vi "a20240618-1.vi"() -> ()   [LabVIEW 2019]
panel:
  out "Array":dbl[](array[numeric])
  out "Numeric 4":dbl
  out "Numeric 3":dbl
  out "Numeric 2":dbl
  in  "stop":bool
  out "Numeric":dbl
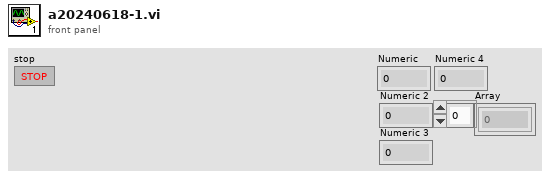
[diagram p1: front panel]
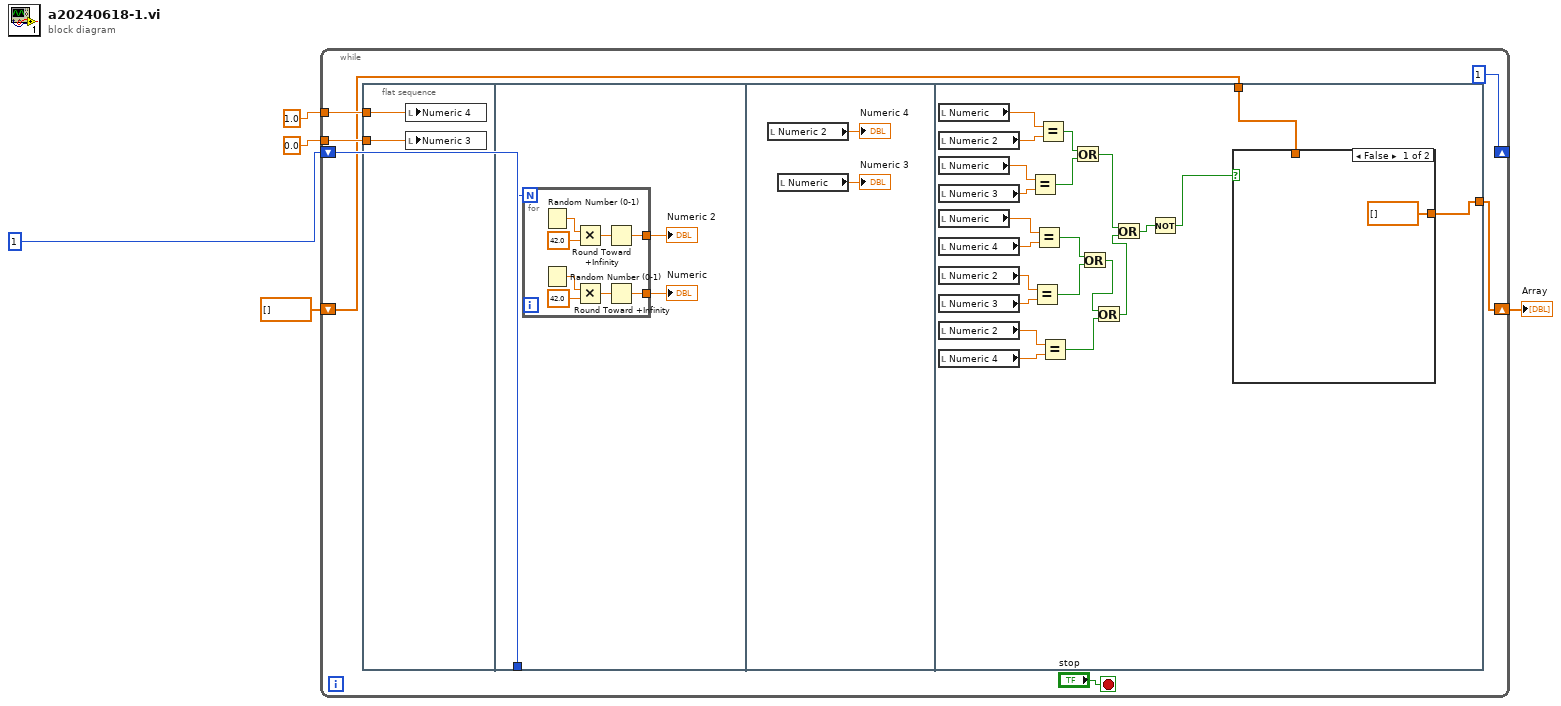
[diagram p0: block diagram]
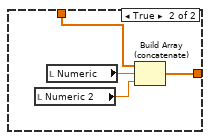
[diagram p2: hidden frame]
diagram:
  n1 = while {
    shift-right: [1] -> _
    shift-left: 1 -> [w11]
    tunnel: 1.0 ("Numeric 3") -> [w10]
    tunnel: 0.0 ("Numeric 3") -> [w9]
    shift-right: [w8] -> w1
    shift-left: dbl[] [] ("Array") -> [w7]
    stop <- "stop" stop-if-true
    n2 = flat-sequence {
      tunnel: w10 -> [w14]
      tunnel: w9 -> [w13]
      tunnel: w11 -> [w15]
      tunnel: [w39] -> w8
      tunnel: w7 -> [w38]
      frame #0 {
        n3 = local write "Numeric 4"(w14) -> ()
        n4 = local write "Numeric 3"(w13) -> ()
      }
      frame #1 {
        n5 = for {
          N: w15 -> [_]
          tunnel: [w22] -> w17
          tunnel: [w18] -> w16
          n6 = Random Number (0-1)() -> (number: 0 to 1=w19:dbl)
          n7 = Random Number (0-1)() -> (number: 0 to 1=w25:dbl)
          n8 = Multiply(x=w19, y=42.0) -> (x*y=w21:dbl)
          n9 = Multiply(x=w25, y=42.0) -> (x*y=w23:dbl)
          n10 = Round Toward +Infinity(x=w21) -> (ceil(x): smallest int >= x=w18:dbl)
          n11 = Round Toward +Infinity(x=w23) -> (ceil(x): smallest int >= x=w22:dbl)
        }
        "Numeric" <- w17
        "Numeric 2" <- w16
      }
      frame #2 {
        n12 = local read "Numeric 2"() -> (→"Numeric 4":dbl)
        n13 = local read "Numeric"() -> (→"Numeric 3":dbl)
      }
      frame #3 {
        n14 = local read "Numeric"() -> (w49:dbl)
        n15 = local read "Numeric 2"() -> (w48:dbl)
        n16 = local read "Numeric"() -> (w46:dbl)
        n17 = local read "Numeric 3"() -> (w47:dbl)
        n18 = local read "Numeric"() -> (w45:dbl)
        n19 = local read "Numeric 4"() -> (w44:dbl)
        n20 = local read "Numeric 2"() -> (w43:dbl)
        n21 = local read "Numeric 3"() -> (w42:dbl)
        n22 = local read "Numeric 2"() -> (w40:dbl)
        n23 = local read "Numeric 4"() -> (w41:dbl)
        n24 = Equal?(x=w46, y=w47) -> (x = y?=w36:bool)
        n25 = Equal?(x=w43, y=w42) -> (x = y?=w34:bool)
        n26 = Equal?(x=w45, y=w44) -> (x = y?=w35:bool)
        n27 = Equal?(x=w49, y=w48) -> (x = y?=w37:bool)
        n28 = Equal?(x=w40, y=w41) -> (x = y?=w33:bool)
        n29 = Or(x=w37, y=w36) -> (x .or. y?=w31:bool)
        n30 = Or(x=w35, y=w34) -> (x .or. y?=w32:bool)
        n31 = Or(x=w32, y=w33) -> (x .or. y?=w30:bool)
        n32 = Or(x=w31, y=w30) -> (x .or. y?=w29:bool)
        n33 = Not(x=w29) -> (.not. x?=w28:bool)
        n34 = case shown="False" w28 {
          tunnel: [dbl[] [] w54] -> w39
          tunnel: w38 -> [_ w51]
          frame False {
          }
          frame True {
            n35 = local read "Numeric 2"() -> (w52:dbl)
            n36 = local read "Numeric"() -> (w53:dbl)
            n37 = Build Array (concatenate)(w51, w53, w52) -> (w54:dbl[])
          }
        }
      }
    }
  }
  "Array" <- w1
